vi "Voltage and resistance setpoint loop.vi"(1 "Resistance setpoint Loop ID":T1, 2 "Voltage setpoint loop ID":T1, 11 "error in (no error)":errorcluster) -> ()   [LabVIEW 2011]
uses:
  Application Structure/Loop ID.ctl
  PCP interface/High Level/PCP High Level Commands.ctl
  PCP interface/High Level/PCP High Level Telegram.ctl
  Application Structure/QSM State List.ctl
  emi Lib/System 01/0 - General/App/Loop control 2/Private/_emi_ SMLoop start condition.vi
  emi Lib/System 01/0 - General/App/Loop control 2/Private/_emi_ SMLoop Error Check.vi
  emi Lib/Basic/0 - General/Error/emi_Is Error.vi
  emi Lib/System 01/0 - General/App/Loop control 2/Private/_emi_SMLoop Register new.vi
  emi Lib/System 01/0 - General/S&E reporting/emi_Send S&E Error message.vi
  emi Lib/Basic/0 - General/Error/emi_ Is Error state.vi
  emi Lib/System 01/0 - General/emi_Read System ID.vi
  emi Lib/System 01/0 - General/App/Loop control/Private/_emi_GFV Loop Linking.vi
  emi Lib/System 01/0 - General/App/Loop control/Private/_emi_GFV Loop Enable.vi
  emi Lib/System 01/0 - General/App/Loop control 2/Private/_emi_ SMLoop Restart.vi
  emi Lib/System 01/0 - General/App/Private/_emi_GFV App Close.vi
  emi Lib/System 01/0 - General/App/Loop control 2/Private/_emi_ SMLoop Restart Counter.vi
  emi Lib/System 01/0 - General/App/Loop control/Private/_emi_GFV Loop Running.vi
  emi Lib/System 01/0 - General/Private/_emi_GFV System ID.vi
  emi Lib/System 01/0 - General/S&E reporting/Private/_emi_S&E Q Generator.vi
  <vilib>/Utility/error.llb/Clear Errors.vi
  emi Lib/System 01/0 - General/App/Loop control/Private/_emi_GFV stop a loop so it can reset.vi
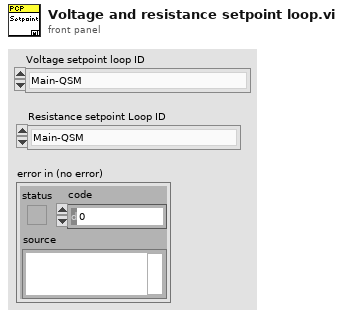
[diagram p1: front panel]
types:
  T1 = typedef "Loop ID.ctl" = enum16{"Main-QSM", "Main-Dialog", "Main-Ind Upd", "Main-Graph Upd", "Main-Debug", "Main-DebugW1", "Main-DebugW2", "Main-SE Handler", "Interface-PCP", "Interface-CANbus", "Interface-Modem", "Var Handling-Beat", "Var Handling-From PCP", "Var Handling-File storage", "Var Handling-From Simulator", "GUI-GrphW Mast", "GUI-GrphW Slav", "SIM-Tool W1", "SIM-Tool W2", "Alm-Sound", "LEIN-motor", "Tool data gatherer Qer", "Tool Data LEIN STAT2 dekoder", "Indicator Value Update", "Tool STAT2 dedicated reader", "Tool ID handler", "Detail View L1", "Detail View L2", "Main display enable view", "Sequence runner", "Voltage setpoint", "Resistance setpoint", "Stroker Wizard L1", "Stroker Wizard L2", "Alarm Handling", "Annotations Tip Strip", "Magna Interface", "Modem Status", "Var Handling - Modem Status", "Power interface detector"}
  T2 = typedef "PCP High Level Commands.ctl" = enum16{"HVPSU HV ON", "HVPSU HV OFF", "PCP PC", "PCP Local", "Update Motor Voltage", "Update Cable Resistance", "Final Motor Voltage", "Final Resistance"}
  T3 = typedef "PCP High Level Telegram.ctl" = cluster{"PCP":T2, "SP":dbl}
  T4 = typedef "QSM State List.ctl" = enum16{"Idle", "Init <<<Start>>>", "Init Reg Controlers", "Init Stroker Ref FGV", "Init Driller Ref FGV", "Init Tractor Ref FGV", "Init All loops", "Init Mem Ctls", "Init GUI", "Init<<<End>>>", "Show options", "Options updated", "Show User Dialog", "User Updated", "Show About", "Show Help", "Debug Visibility", "End Application", "Mem Ctls", "Mem Graphs", "Post", "-------------", "Dialog Common Analog", "Chart Init", "Chart Var Selector Rings init", "Chart Read Settings from INI", "Chart Clear", "Chart Selection Changed", "Chart Time Changed", "Graph Dialog Show", "Annotation, New", "Annotation Created", "PCP CMD", "Show Welcome screen", "Dialog Tool analog", "Update PCP resistance", "Tool CMD", "Chart single autoscale", "Tool connenction state", "Show detailed view", "Sequences updated", "Show stroker wizard", "Change tool", "Reset Telemetry", "Update control units", "Stop Logging", "Start New Loggfile", "Log Init", "Copy INI files"}
  T5 = typedef "_emi_ SMLoop sates.ctl" = enum16{"Init", "Standby", "Start", "Normal Operation", "Stop", "Error Handling", "End", "Post"}
  T6 = cluster{"Ongoing":bool, "Setpoint table":dbl[], "Previous value":dbl}
  T7 = typedef "Options  All pages and custom.ctl" = cluster{"P 1 (App)":T8, "P 2":T9, "P 3":T10, "P 4":T13, "P 5":T18, "P 6 (Err)":T19, "P 7 (Expert)":T20, "P 8 (Depth)":T22, "C 1":T23, "C 2":T24}
  T8 = typedef "Options Page 1 (App).ctl" = cluster{"Result files":path, "PCP Interface":string, "Tractor/Stroker Interface":string, "Tractor Interface":string, "Modem Status Interface":string, "Audible Alarm":bool, "Force alarm on Technical":bool, "Force alarm on HH":bool, "Force alarm on LL":bool, "Force alarm on H":bool, "Force alarm on L":bool}
  T9 = typedef "Options Page 2.ctl" = cluster{"Solenoid & Relay latching time":u16, "Tractor relay 1":dbl, "Tractor relay 2":dbl, "Tractor Solenoid limit":dbl}
  T10 = typedef "Options Page 3.ctl" = cluster{"Min resistance":dbl, "Max resistance":dbl, "Head voltage range":T11, "Max voltage jump":dbl, "Maximum resistance change":dbl, "Start Telemetry Voltage":dbl, "Start Telemetry Timeout":dbl, "Start Motor Voltage":dbl, "Stop Motor Voltage":dbl, "Pass Mode Warning Voltage":dbl, "Relay Switch Voltage":dbl, "Relay Status Loss Voltage":dbl, "Samples to average":i32, "PSU type DO NOT USE":T12, "Magna OVP":dbl, "Magna Current Limit":dbl}
  T11 = typedef "PCP type List.ctl" = enum16{"0 - 350V", "0 - 450V", "0 - 600V"}
  T12 = typedef "PSU Type.ctl" = enum16{"Unipower", "Magna 8.3A", "Magna 12A", "None"}
  T13 = typedef "Options Page 4.ctl" = cluster{"Solenoid & Relay latching time":u16, "Stroker relay 1":dbl, "Stroker Relay 2":dbl, "Stroker Solenoid limit":dbl, "Force det.":T14, "Stroke force lim.":dbl, "Anchor Enabled Pressure":dbl, "Tacometer puls":dbl, "Default anchor behavior":T15, "Default stroker behavior":T16, "Default stroker force limit (tonne)":dbl, "Slips Size":T17}
  T14 = typedef "Stroke force selector.ctl" = enum16{"Stroke in = node 1", "Strok out = node 1"}
  T15 = typedef "Default anchor behavior.ctl" = enum16{"Do nothing", "Set Anchor", "Release Anchor"}
  T16 = typedef "Default stroker behavior.ctl" = enum16{"Do nothing", "Stop", "Go Out", "Go In"}
  T17 = typedef "Slips Type Radio.ctl" = enum32{"No Selection", "338 MRS", "3,9 MRS"}
  T18 = typedef "Options Page 5.ctl" = cluster{"Solenoid & Relay latching time":u16, "Driller relay 1":dbl, "Driller Relay 2":dbl, "Driller  Solenoid limit":dbl}
  T19 = typedef "Options Page 6 (Err).ctl" = cluster{"Error and event files":path}
  T20 = typedef "Options Page 7 (Expert).ctl" = cluster{"Show Debug":bool, "Log debug messages":bool, "Additional debug messages":bool, "Start Beagle with Simulator data":bool, "Workshop mode":bool, "Modem baud":u16, "enumCANCOM":bool, "Modem sim":T21, "Telemetry Timeout Disable":i32, "Buffer size":i32, "Upd regular data":bool, "Cable comp":cluster{"VMOD1 Voltage(V)":dbl, "VMOD2 Voltage(V)":dbl}}
  T21 = typedef "Modem simulation setup.ctl" = cluster{"Modem dealay sim":bool, "Sim baud Tx":u16, "Bit Error fraction Tx":dbl, "Sim baud Rx":u16, "Bit Error fraction Rx":dbl}
  T22 = typedef "Options Page 8 (Depth).ctl" = cluster{"Winch Spool Circumference":dbl, "Winch Pulses per Revolution":dbl, "Current Depth":dbl}
  T23 = typedef "Options Custom 1.ctl" = cluster{"Depth Updated":bool, "Depth Offset":dbl}
  T24 = typedef "Options Custom 2.ctl" = cluster{"Placeholder":bool}
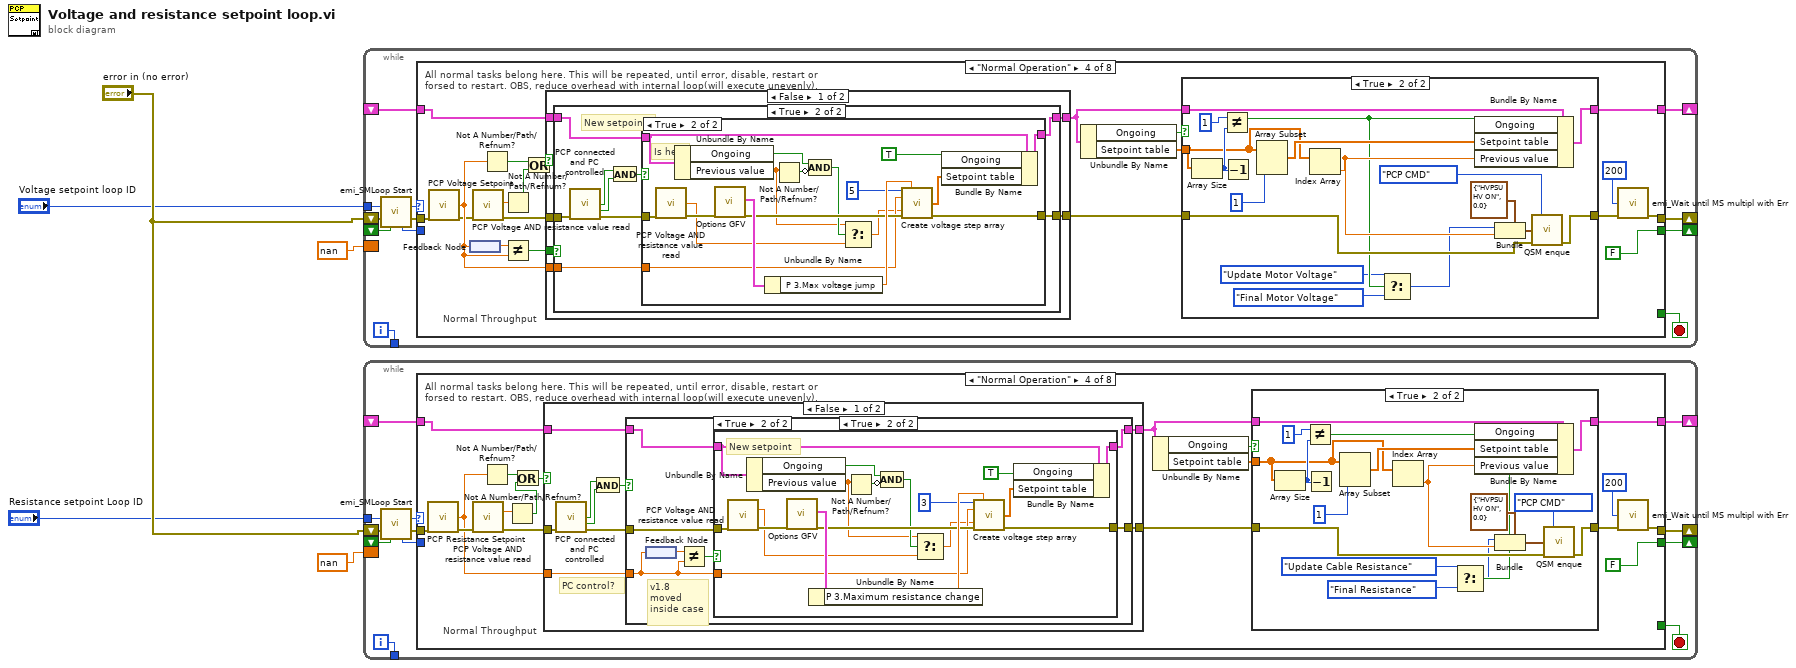
[diagram p0: block diagram]
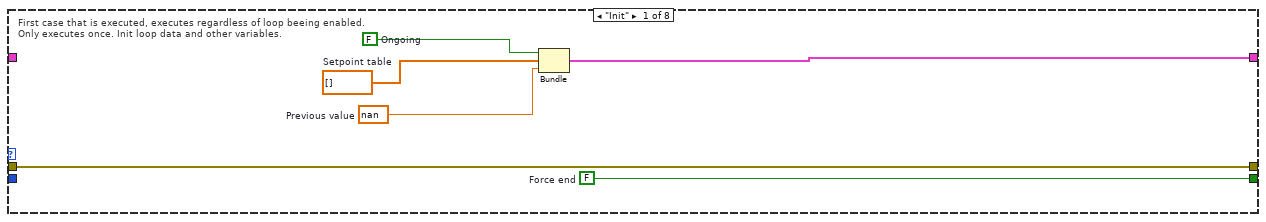
[diagram p2: hidden frame]
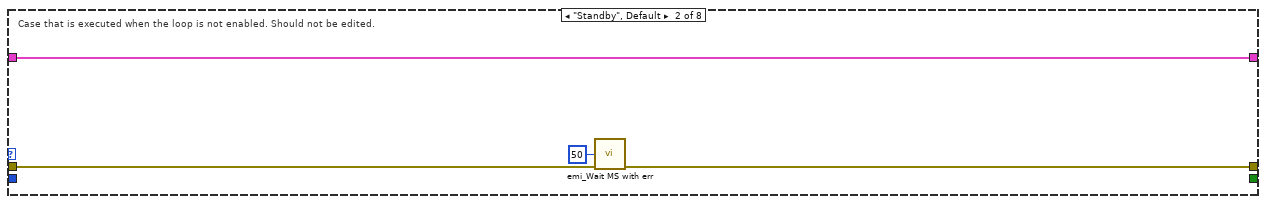
[diagram p3: hidden frame]
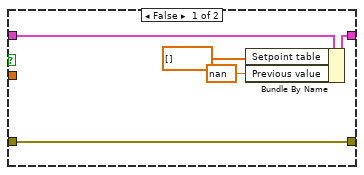
[diagram p5: hidden frame]
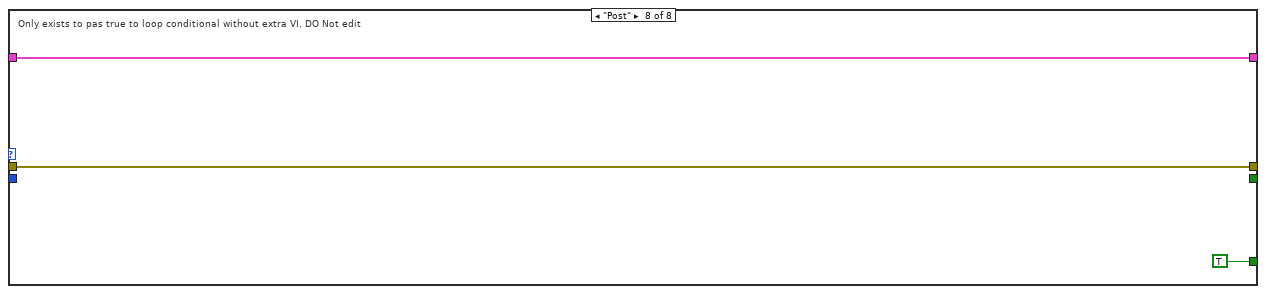
[diagram p12: hidden frame]
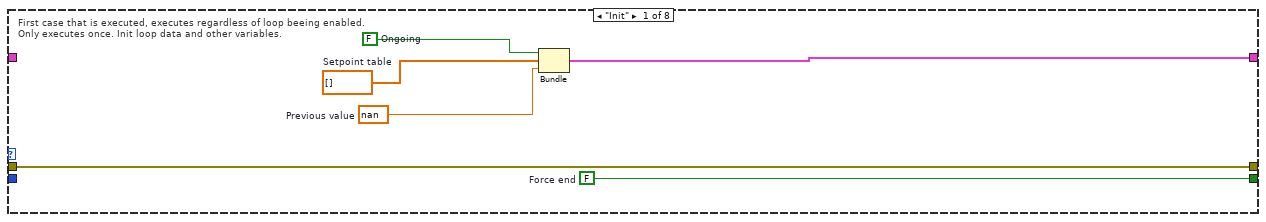
[diagram p13: hidden frame]
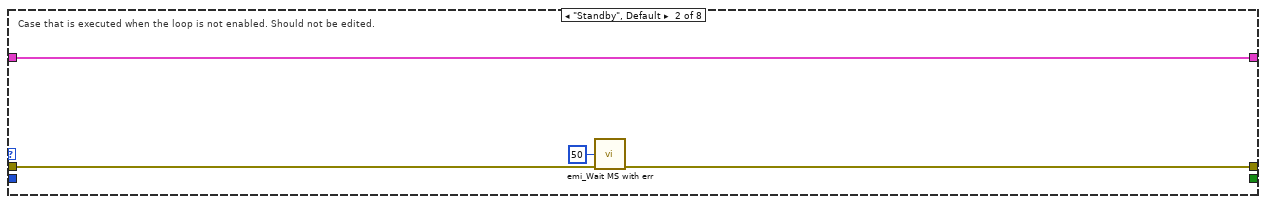
[diagram p14: hidden frame]
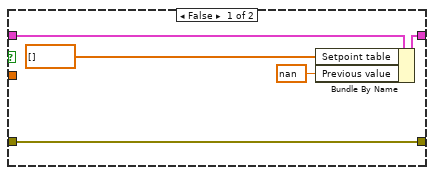
[diagram p16: hidden frame]
diagram:
  n1 = while {
    shift-right: [w17] -> _
    shift-left: _ -> [w13]
    shift-right: [w15] -> _
    shift-left: "error in (no error)" -> [w11]
    tunnel: [w14] -> _
    shift-right: [w12] -> _
    shift-left: _ -> [w7]
    tunnel: "Voltage setpoint loop ID" -> [w8]
    border: nan -> [_]
    i -> [w14]
    stop <- w16 stop-if-true
    n2 = call "emi_SMLoop Start.vi"("Loop ID"=w8, "error in (no error)"=w11, "Force Stop(F)"=w7) -> ("Loop command"=w9:T5, "error out"=w10:errorcluster, "Loop ID out"=w6:i32)  [unwired: 10 in]
    n3 = case shown="\"Normal Operation\"" w9 {
      tunnel: [w22 w24 w28 w38 w111 w114 w115 w118] -> w17
      tunnel: [_ _ _ _ _ _ _ TRUE] -> w16
      tunnel: w10 -> [w23 w26 w29 w48 w112 w113 w116 w119]
      tunnel: [w23 w25 w29 w47 w112 w113 w116 w119] -> w15
      tunnel: w13 -> [_ w24 w28 w42 w111 w114 w115 w118]
      tunnel: [w20 _ _ FALSE ("Force End") _ _ _ _] -> w12
      tunnel: w6 -> [_ _ _ _ _ _ _ _]
      frame "Init" {
        w18 = nan  # Previous value
        w19 = dbl[] []  # Setpoint table
        w20 = FALSE  # Force end
        w21 = FALSE  # Ongoing
        # "First case that is executed, executes regardless of loop beeing enabled.\nOnly executes once. Init loop data and other variables."
        n4 = Bundle("Ongoing"=w21, "Setpoint table"=w19, "Previous value"=w18) -> (w22:T6)  [unwired: 1 in]
      }
      frame "Standby", Default {
        # "Case that is executed when the loop is not enabled. Should not be edited."
        n5 = call "emi_Wait MS with err.vi"("milliseconds to wait(0)"=u32 50, "error in (no error)"=w26) -> ("error out"=w25:errorcluster)  [unwired: 13 in]
      }
      frame "Start" {
        # "Start or restart the loop. Should perform any init code. \nOpen channel and so on. Will perform each time the system is restarted."
      }
      frame "Normal Operation" {
        # "Normal Throughput"
        # "All normal tasks belong here. This will be repeated, until error, disable, restart or\nforsed to restart. OBS, reduce overhead with internal loop(will execute unevenly)."
        n6 = call "PCP Voltage Setpoint.vi"("error in (no error)"=w48) -> ("PCP setpoint"=w41:dbl, "error out"=w34:errorcluster)  [unwired: 13 in]
        n7 = feedback-in #1(w41) -> ()
        n8 = feedback #1() -> (w44:dbl)
        n9 = call "PCP Voltage AND resistance value read.vi"("error in (no error)"=w34) -> ("PCP voltage out"=w32:dbl, "error out"=w33:errorcluster)  [unwired: 12 in, 1 out]
        n10 = Not A Number/Path/Refnum?(number/path/refnum=w41) -> (NaN/Path/Refnum?=w45:bool)
        n11 = Not A Number/Path/Refnum?(number/path/refnum=w32) -> (NaN/Path/Refnum?=w30:bool)
        n12 = Not Equal?(x=w44, y=w41) -> (x != y?=w43:bool)
        n13 = Or(x=w45, y=w30) -> (x .or. y?=w31:bool)
        n14 = case shown="False" w31 {
          tunnel: [w72 w110] -> w35
          tunnel: w33 -> [w76 w110]
          tunnel: w43 -> [w77 _]
          tunnel: w42 -> [w75 w109]
          tunnel: [w74 w109] -> w39
          tunnel: w41 -> [w73 _]
          frame False {
            n15 = case shown="True" w77 {
              tunnel: w76 -> [w78 w88]
              tunnel: w75 -> [w79 w85]
              tunnel: [w79 w84] -> w74
              tunnel: w73 -> [_ w82]
              tunnel: [w78 w81] -> w72
              frame False {
              }
              frame True {
                # "New setpoint"
                n16 = call "PCP connected and PC controlled.vi"("error in (no error)"=w88) -> ("PCP connected out"=w86:bool, "PCP PC controlled out"=w87:bool, "error out"=w83:errorcluster)  [unwired: 12 in]
                n17 = And(x=w86, y=w87) -> (x .and. y?=w80:bool)
                n18 = case shown="True" w80 {
                  tunnel: w85 -> [w90 w99]
                  tunnel: [w90 w101] -> w84
                  tunnel: w83 -> [w89 w108]
                  tunnel: w82 -> [_ w92]
                  tunnel: [w89 w102] -> w81
                  frame False {
                    # "Not availøable for funckin with so disregard."
                  }
                  frame True {
                    # "Is here"
                    n19 = call "PCP Voltage AND resistance value read.vi"("error in (no error)"=w108) -> ("PCP voltage out"=w104:dbl, "error out"=w107:errorcluster)  [unwired: 12 in, 1 out]
                    n20 = Unbundle By Name(w99) -> ("Ongoing"=w98:bool, "Previous value"=w95:dbl)
                    n21 = call "Options GFV.vi"("error in (no error)"=w107) -> ("Options"=w106:T7, "error out"=w103:errorcluster)  [unwired: 16 in, 1 out]
                    n22 = Unbundle By Name(w106) -> ("P 3.Max voltage jump"=w105:dbl)
                    n23 = Not A Number/Path/Refnum?(number/path/refnum=w95) -> (NaN/Path/Refnum?=w97:bool)
                    n24 = Compound Arithmetic op=AND(w98, invert w97) -> (w96:bool)
                    n25 = Select(t=w95, s=w96, f=w104) -> (s? t:f=w91:dbl)
                    n26 = call "Create voltage step array.vi"("Min numb steps"=5, "Max voltage jump"=w105, "Setpoint"=w92, "Current/ last  value"=w91, "error in (no error)"=w103) -> ("Array"=w93:dbl[], "error out"=w102:errorcluster)  [unwired: 9 in]
                    n27 = Bundle By Name(cluster=w99, "Ongoing"=TRUE, "Setpoint table"=w93) -> (w101:T6)
                  }
                }
              }
            }
          }
          frame True {
            # "Not really started"
          }
        }
        n28 = Unbundle By Name(w39) -> ("Ongoing"=w40:bool, "Setpoint table"=w37:dbl[])
        n29 = case shown="True" w40 {
          tunnel: w39 -> [w54 w71]
          tunnel: [w53 w66] -> w38
          tunnel: w37 -> [_ w67]
          tunnel: [w51 w61] -> w36
          tunnel: w35 -> [w51 w62]
          frame False {
            n30 = Bundle By Name(cluster=w54, "Setpoint table"=dbl[] [], "Previous value"=nan) -> (w53:T6)
          }
          frame True {
            n31 = Array Size(array=w67) -> (size(s)=w70:i32)
            n32 = Not Equal?(x=1, y=w70) -> (x != y?=w58:bool)
            n33 = Decrement(x=w70) -> ()  [unwired: 1 out]
            n34 = Array Subset(array=w67, index=1) -> (w68:dbl[])  [unwired: 1 in]
            n35 = Index Array(array=w67) -> (element=w60:dbl)  [unwired: 1 in]
            n36 = Select(t=PCP_High_Level_Commands."Update Motor Voltage" ("PCP"), s=w58, f=PCP_High_Level_Commands."Final Motor Voltage" ("PCP")) -> (s? t:f=w55:T2)
            n37 = Bundle By Name(cluster=w71, "Ongoing"=w58, "Setpoint table"=w68, "Previous value"=w60) -> (w66:T6)
            n38 = Bundle(cluster=T3 {"PCP"=enum."HVPSU HV ON", "SP"=0.0} ("PCP beskjed"), "PCP"=w55, "SP"=w60) -> (w65:T3)
            n39 = call "QSM enque.vi"("State"=QSM_State_List."PCP CMD", "Value"=w65, "error in"=w62) -> ("error out"=w61:errorcluster)  [unwired: 12 in]
          }
        }
        n40 = call "emi_Wait until MS multipl with Err.vi"("millisecond multiple(0)"=u32 200, "error in (no error)"=w36) -> ("error out"=w47:errorcluster)  [unwired: 13 in]
      }
      frame "Stop" {
        # "Stop the loop. May be restarted later. Close interfaces and the like"
      }
      frame "Error Handling" {
        # "Loop automaticaly returns here after error is found. If error is cleared, \nLoop wil continue as normal(if was operative when error."
      }
      frame "End" {
        # "Only executes at application end has. Should performa any action the loop \nneeds to finnish. Executes only once."
      }
      frame "Post" {
        # "Only exists to pas true to loop conditional without extra VI. DO Not edit"
      }
    }
  }
  n41 = while {
    shift-right: [w131] -> _
    shift-left: _ -> [w127]
    shift-right: [w129] -> _
    shift-left: "error in (no error)" -> [w125]
    tunnel: [w128] -> _
    shift-right: [w126] -> _
    shift-left: _ -> [w121]
    tunnel: "Resistance setpoint Loop ID" -> [w122]
    border: nan -> [_]
    i -> [w128]
    stop <- w130 stop-if-true
    n42 = call "emi_SMLoop Start.vi"("Loop ID"=w122, "error in (no error)"=w125, "Force Stop(F)"=w121) -> ("Loop command"=w123:T5, "error out"=w124:errorcluster, "Loop ID out"=w120:i32)  [unwired: 10 in]
    n43 = case shown="\"Normal Operation\"" w123 {
      tunnel: [w136 w138 w142 w154 w224 w227 w228 w231] -> w131
      tunnel: [_ _ _ _ _ _ _ TRUE] -> w130
      tunnel: w124 -> [w137 w140 w143 w146 w225 w226 w229 w232]
      tunnel: [w137 w139 w143 w160 w225 w226 w229 w232] -> w129
      tunnel: w127 -> [_ w138 w142 w157 w224 w227 w228 w231]
      tunnel: [w134 _ _ FALSE ("Force End") _ _ _ _] -> w126
      tunnel: w120 -> [_ _ _ _ _ _ _ _]
      frame "Init" {
        w132 = nan  # Previous value
        w133 = dbl[] []  # Setpoint table
        w134 = FALSE  # Force end
        w135 = FALSE  # Ongoing
        # "First case that is executed, executes regardless of loop beeing enabled.\nOnly executes once. Init loop data and other variables."
        n44 = Bundle("Ongoing"=w135, "Setpoint table"=w133, "Previous value"=w132) -> (w136:T6)  [unwired: 1 in]
      }
      frame "Standby", Default {
        # "Case that is executed when the loop is not enabled. Should not be edited."
        n45 = call "emi_Wait MS with err.vi"("milliseconds to wait(0)"=u32 50, "error in (no error)"=w140) -> ("error out"=w139:errorcluster)  [unwired: 13 in]
      }
      frame "Start" {
        # "Start or restart the loop. Should perform any init code. \nOpen channel and so on. Will perform each time the system is restarted."
      }
      frame "Normal Operation" {
        # "Normal Throughput"
        # "All normal tasks belong here. This will be repeated, until error, disable, restart or\nforsed to restart. OBS, reduce overhead with internal loop(will execute unevenly)."
        n46 = call "PCP Resistance Setpoint.vi"("error in (no error)"=w146) -> ("PCP RES  setpoint"=w144:dbl, "error out"=w145:errorcluster)  [unwired: 13 in]
        n47 = call "PCP Voltage AND resistance value read.vi"("error in (no error)"=w145) -> ("PCP resistance out 2"=w148:dbl, "error out"=w150:errorcluster)  [unwired: 12 in, 1 out]
        n48 = Not A Number/Path/Refnum?(number/path/refnum=w144) -> (NaN/Path/Refnum?=w158:bool)
        n49 = Not A Number/Path/Refnum?(number/path/refnum=w148) -> (NaN/Path/Refnum?=w147:bool)
        n50 = Or(x=w158, y=w147) -> (x .or. y?=w149:bool)
        n51 = case shown="False" w149 {
          tunnel: [w190 w223] -> w151
          tunnel: w150 -> [w186 w223]
          tunnel: w157 -> [w192 w222]
          tunnel: [w191 w222] -> w155
          tunnel: w144 -> [w189 _]
          frame False {
            # "PC control?"
            n52 = call "PCP connected and PC controlled.vi"("error in (no error)"=w186) -> ("PCP connected out"=w188:bool, "PCP PC controlled out"=w187:bool, "error out"=w185:errorcluster)  [unwired: 12 in]
            n53 = And(x=w188, y=w187) -> (x .and. y?=w184:bool)
            n54 = case shown="True" w184 {
              tunnel: w185 -> [w193 w195]
              tunnel: w192 -> [w194 w201]
              tunnel: [w194 w200] -> w191
              tunnel: w189 -> [_ w197]
              tunnel: [w193 w199] -> w190
              frame False {
              }
              frame True {
                # "v1.8\nmoved\ninside case"
                n55 = feedback #2() -> (w198:dbl)
                n56 = feedback-in #2(w197) -> ()
                n57 = Not Equal?(x=w198, y=w197) -> (x != y?=w196:bool)
                n58 = case shown="True" w196 {
                  tunnel: w201 -> [w203 w213]
                  tunnel: [w203 w215] -> w200
                  tunnel: w195 -> [w202 w221]
                  tunnel: w197 -> [_ w206]
                  tunnel: [w202 w216] -> w199
                  frame False {
                    # "Not availøable for funckin with so disregard."
                  }
                  frame True {
                    # "New setpoint"
                    n59 = call "PCP Voltage AND resistance value read.vi"("error in (no error)"=w221) -> ("PCP resistance out 2"=w204:dbl, "error out"=w220:errorcluster)  [unwired: 12 in, 1 out]
                    n60 = Unbundle By Name(w213) -> ("Ongoing"=w212:bool, "Previous value"=w209:dbl)
                    n61 = call "Options GFV.vi"("error in (no error)"=w220) -> ("Options"=w219:T7, "error out"=w217:errorcluster)  [unwired: 16 in, 1 out]
                    n62 = Unbundle By Name(w219) -> ("P 3.Maximum resistance change"=w218:dbl)
                    n63 = Not A Number/Path/Refnum?(number/path/refnum=w209) -> (NaN/Path/Refnum?=w211:bool)
                    n64 = Compound Arithmetic op=AND(w212, invert w211) -> (w210:bool)
                    n65 = Select(t=w209, s=w210, f=w204) -> (s? t:f=w205:dbl)
                    n66 = call "Create voltage step array.vi"("Min numb steps"=3, "Max voltage jump"=w218, "Setpoint"=w206, "Current/ last  value"=w205, "error in (no error)"=w217) -> ("Array"=w207:dbl[], "error out"=w216:errorcluster)  [unwired: 9 in]
                    n67 = Bundle By Name(cluster=w213, "Ongoing"=TRUE, "Setpoint table"=w207) -> (w215:T6)
                  }
                }
              }
            }
          }
          frame True {
            # "Not really started"
          }
        }
        n68 = Unbundle By Name(w155) -> ("Ongoing"=w156:bool, "Setpoint table"=w153:dbl[])
        n69 = case shown="True" w156 {
          tunnel: w155 -> [w166 w183]
          tunnel: [w165 w178] -> w154
          tunnel: w153 -> [_ w179]
          tunnel: [w163 w173] -> w152
          tunnel: w151 -> [w163 w174]
          frame False {
            n70 = Bundle By Name(cluster=w166, "Setpoint table"=dbl[] [], "Previous value"=nan) -> (w165:T6)
          }
          frame True {
            n71 = Array Size(array=w179) -> (size(s)=w182:i32)
            n72 = Not Equal?(x=1, y=w182) -> (x != y?=w170:bool)
            n73 = Decrement(x=w182) -> ()  [unwired: 1 out]
            n74 = Array Subset(array=w179, index=1) -> (w180:dbl[])  [unwired: 1 in]
            n75 = Index Array(array=w179) -> (element=w172:dbl)  [unwired: 1 in]
            n76 = Select(t=PCP_High_Level_Commands."Update Cable Resistance" ("PCP"), s=w170, f=PCP_High_Level_Commands."Final Resistance" ("PCP")) -> (s? t:f=w167:T2)
            n77 = Bundle By Name(cluster=w183, "Ongoing"=w170, "Setpoint table"=w180, "Previous value"=w172) -> (w178:T6)
            n78 = Bundle(cluster=T3 {"PCP"=enum."HVPSU HV ON", "SP"=0.0} ("PCP beskjed"), "PCP"=w167, "SP"=w172) -> (w177:T3)
            n79 = call "QSM enque.vi"("State"=QSM_State_List."PCP CMD", "Value"=w177, "error in"=w174) -> ("error out"=w173:errorcluster)  [unwired: 12 in]
          }
        }
        n80 = call "emi_Wait until MS multipl with Err.vi"("millisecond multiple(0)"=u32 200, "error in (no error)"=w152) -> ("error out"=w160:errorcluster)  [unwired: 13 in]
      }
      frame "Stop" {
        # "Stop the loop. May be restarted later. Close interfaces and the like"
      }
      frame "Error Handling" {
        # "Loop automaticaly returns here after error is found. If error is cleared, \nLoop wil continue as normal(if was operative when error."
      }
      frame "End" {
        # "Only executes at application end has. Should performa any action the loop \nneeds to finnish. Executes only once."
      }
      frame "Post" {
        # "Only exists to pas true to loop conditional without extra VI. DO Not edit"
      }
    }
  }
